vi "Init Tokenizer.vi"(10 "Policy":T1, 11 "Input":string) -> (3 "Tokenizer":T2)   [LabVIEW 2020, in "Stream.lvlib" / "URLPattern.lvclass"]
uses:
  URLPattern.lvclass
  Token Type.ctl
  Token.ctl
  Tokenizer.ctl
  Tokenize Policy.ctl
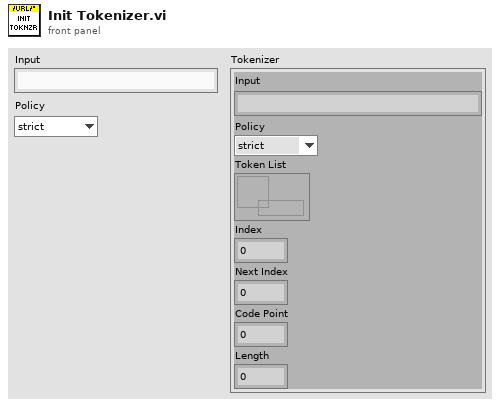
[diagram p1: front panel]
types:
  T1 = typedef "Stream.lvlib/URLPattern.lvclass/Tokenize Policy.ctl" = enum16{"strict", "lenient"}
  T2 = typedef "Stream.lvlib/URLPattern.lvclass/Tokenizer.ctl" = cluster{"Input":string, "Policy":T1, "Token List":refnum<queue>, "Index":i32, "Next Index":i32, "Code Point":u32, "Length":i32}
  T3 = typedef "Stream.lvlib/URLPattern.lvclass/Token.ctl" = cluster{"Type":T4, "Index":i32, "Value":string}
  T4 = typedef "Stream.lvlib/URLPattern.lvclass/Token Type.ctl" = enum16{"invalid-char", "open", "close", "regexp", "name", "char", "escaped-char", "other-modifier", "asterisk", "end"}
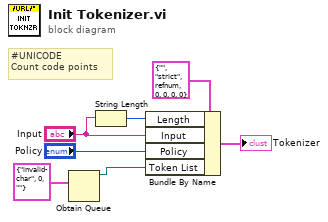
[diagram p0: block diagram]
diagram:
  # "#UNICODE\nCount code points"
  n1 = Obtain Queue(element data type=T3 {"Type"=enum."invalid-char", "Index"=0, "Value"=""} ("Token")) -> (queue out=w3:refnum<queue>)  [unwired: 4 in, 2 out]
  n2 = String Length(string="Input") -> (length=w1:i32)
  n3 = Bundle By Name(cluster=T2 {"Input"="", "Policy"=enum."strict", "Token List"=refnum, "Index"=0, "Next Index"=0, "Code Point"=0, "Length"=0} ("Tokenizer"), "Length"=w1, "Input"="Input", "Policy"="Policy", "Token List"=w3) -> (→"Tokenizer":T2)
